vi "PCAN_Terminal.vi"() -> ()   [LabVIEW 2023, in "pCANLib.lvlib"]
uses:
  pCANLib.lvlib
panel:
  in  "pathCAN_DLL":path
  out "Array":T1(array[cluster]) {"ID" format="%.0x"}
  out "Version":string
  in  "type":i32(ring) items=["standart", "extended"]
  in  "baud":u16(ring)=20 items=["1M"=20, "500K"=28, "250K"=284, "125K"=796, "100K"=17199, "50K"=18223, "20K"=21295, "10K"=26415, "5K"=32639]
  in  "TPCANMsg To Write":T2 {"ID" format="%x"; "MSGTYPE" items=["STATUS"=128, "EXTENDED"=2, "RTR"=1, "DATA MSG"=0]; "aDATA" format="%x"}
  in  "Write":bool
  out "Last Error":string
  out "TPCANMsg":T2 {"ID" format="%x"; "MSGTYPE" items=["STATUS"=128, "EXTENDED"=2, "RTR"=1, "DATA MSG"=0]; "aDATA" format="%x"}
  in  "stop":bool
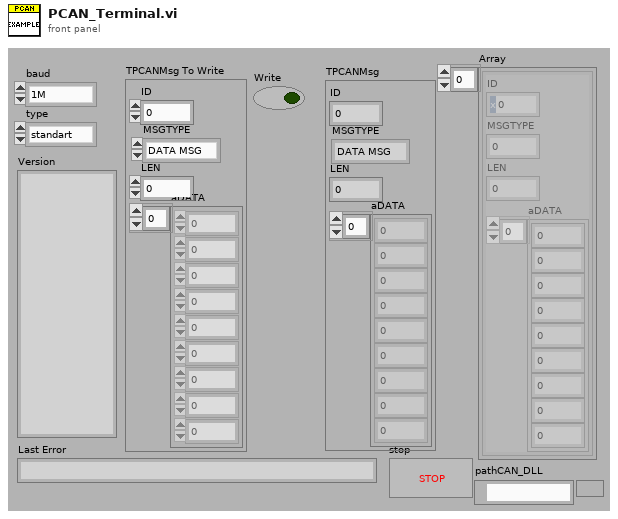
[diagram p1: front panel]
types:
  T1 = cluster{"ID":u32, "MSGTYPE":u8, "LEN":u8, "aDATA":u8[]}[]
  T2 = cluster{"ID":u32, "MSGTYPE":u8, "LEN":u8, "aDATA":u8[]}
  T3 = cluster{"Is Warning":bool, "Is Error":bool, "Message":string}
  T4 = typedef "pCANLib.lvlib/PCAN_ERROR.ctl" = i32
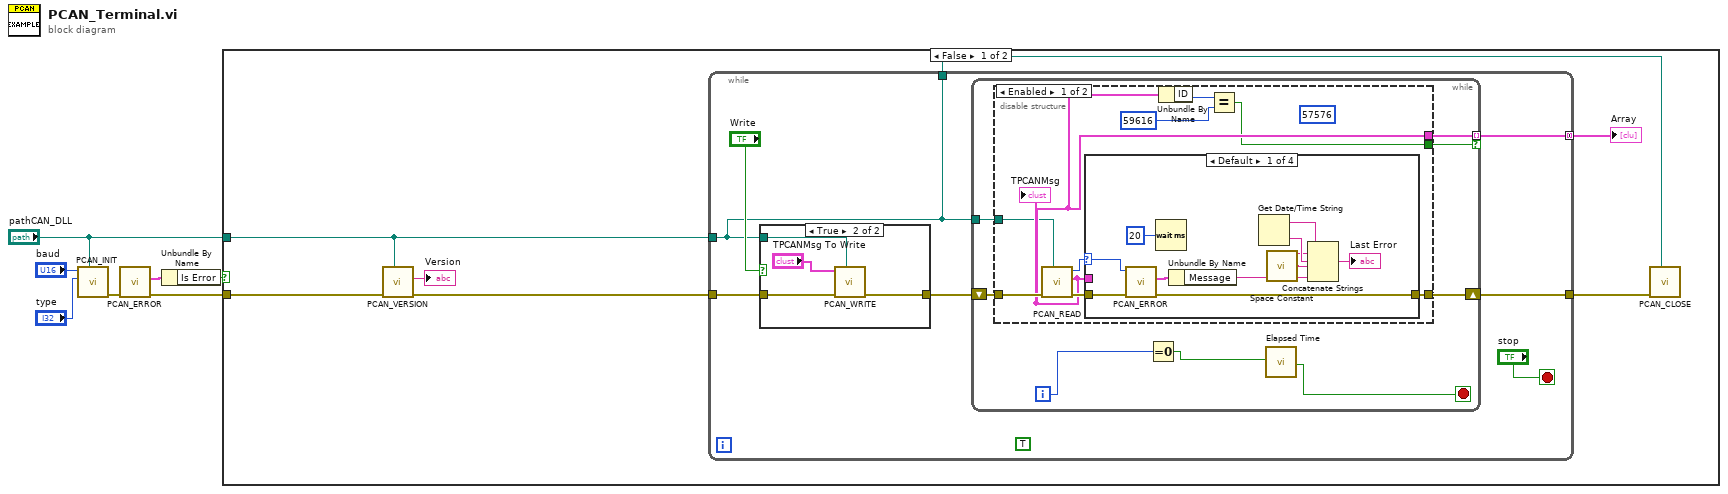
[diagram p0: block diagram]
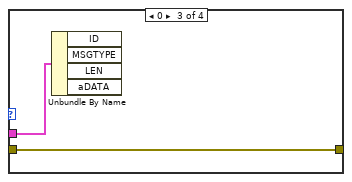
[diagram p3: hidden frame]
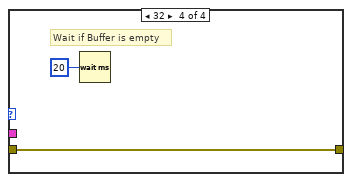
[diagram p4: hidden frame]
diagram:
  n1 = call "PCAN_INIT.vi"("pathCAN_DLL"="pathCAN_DLL", "Msg Type"="type", "BTR0BTR1"="baud") -> ("error out"=w5:errorcluster)  [unwired: 1 in, 7 out]
  n2 = call "PCAN_ERROR.vi"("error in (no error)"=w5) -> ("error out"=w4:errorcluster, "PCAN error"=w3:T3)  [unwired: 1 in, 8 out]
  n3 = Unbundle By Name(w3) -> ("Is Error"=w2:bool)
  n4 = case shown="False" w2 {
    tunnel: w4 -> [w12 _]
    tunnel: "pathCAN_DLL" -> [w9 _]
    frame False {
      n5 = call "PCAN_VERSION.vi"("pathCAN_DLL"=w9, "error in (no error)"=w12) -> ("error out"=w11:errorcluster, "lpszTextBuff"=→"Version":string)  [unwired: 8 out]
      n6 = while {
        tunnel: [w21] -> w14
        tunnel: w11 -> [w18]
        tunnel: [w16] -> w10 mode=concatenating
        tunnel: w9 -> [w15]
        tunnel: [w15] -> w8
        stop <- "stop" stop-if-true
        (unwired) TRUE
        n7 = case shown="True" "Write" {
          tunnel: w18 -> [w54 w58]
          tunnel: [w54 w56] -> w17
          tunnel: w15 -> [_ w55]
          frame False {
          }
          frame True {
            n8 = call "PCAN_WRITE.vi"("pathCAN_DLL"=w55, "error in (no error)"=w58, "TPCANMsg"="TPCANMsg To Write") -> ("error out"=w56:errorcluster)  [unwired: 8 out]
          }
        }
        n9 = while {
          shift-right: [w28] -> w21
          shift-left: w17 -> [w29]
          tunnel: [w24] -> w16 mode=indexing if=w23
          tunnel: w15 -> [w22]
          i -> [w26]
          stop <- w27 stop-if-true
          n10 = disable-structure shown="Enabled" {
            disable-tunnel: w29 -> [w38 _]
            disable-tunnel: [w37 _] -> w28
            disable-tunnel: [w34 _] -> w24
            disable-tunnel: [w31 _] -> w23
            disable-tunnel: w22 -> [w30 _]
            frame Enabled {
              (unwired) u32 57576 ("ID")
              n11 = call "PCAN_READ.vi"("pathCAN_DLL"=w30, "error in (no error)"=w38) -> ("error out"=w35:errorcluster, "TPCANMsg"=w34:T2, "error"=w36:T4)  [unwired: 7 out]
              "TPCANMsg" <- w34
              n12 = case shown="Default" w36 {
                selector: w36 -> [w47 _ _ _]
                tunnel: w34 -> [_ _ w50 _]
                tunnel: w35 -> [w48 w49 w51 w52]
                tunnel: [w46 w49 w51 w52] -> w37
                frame Default {
                  n13 = call "PCAN_ERROR.vi"("error in (no error)"=w48, "Error Code"=w47) -> ("error out"=w46:errorcluster, "PCAN error"=w45:T3)  [unwired: 8 out]
                  n14 = Wait (ms)(milliseconds to wait=u32 20) -> ()  [unwired: 1 out]
                  n15 = Unbundle By Name(w45) -> ("Message"=w40:string)
                  n16 = Get Date/Time String() -> (date string=w43:string, time string=w42:string)  [unwired: 3 out]
                  n17 = call <vilib>:"Space Constant.vi"() -> ("String"=w39:string)
                  n18 = Concatenate Strings(w43, w39, w42, w39, w40) -> (→"Last Error":string)
                }
                frame 59616 {
                }
                frame 0 {
                  n19 = Unbundle By Name(w50) -> ()  [unwired: 4 out]
                }
                frame 32 {
                  # "Wait if Buffer is empty"
                  n20 = Wait (ms)(milliseconds to wait=u32 20) -> ()  [unwired: 1 out]
                }
              }
              n21 = Unbundle By Name(w34) -> ("ID"=w33:u32)
              n22 = Equal?(x=w33, y=u32 59616 ("ID")) -> (x = y?=w31:bool)
            }
            frame Disabled {
            }
          }
          n23 = Equal To 0?(x=w26) -> (x = 0?=w25:bool)
          n24 = call "Elapsed Time"("Reset"=w25) -> ("Time has Elapsed"=w27:bool)  [unwired: 11 in, 7 out]
        }
      }
      "Array" <- w10
      n25 = call "PCAN_CLOSE.vi"("pathCAN_DLL"=w8, "error in (no error)"=w14) -> ()  [unwired: 10 out]
    }
    frame True {
    }
  }
